vi "MKS METER - Error Handler.vi"(8 "error in (no error)":errorcluster, 10 "Channel String":string, 11 "Channel":T1(ring)) -> (0 "error out":errorcluster)   [LabVIEW 2013]
uses:
  <vilib>/Utility/error.llb/DialogType.ctl
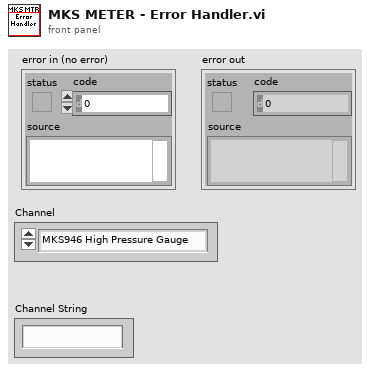
[diagram p1: front panel]
types:
  T1 = enum16{"MKS946 High Pressure Gauge", "MKS946 Separator Flow", "MKS946 Target Cavity Flow", "MKS670 Low Pressure Gauge"}
  T2 = typedef "DialogType.ctl" = u16
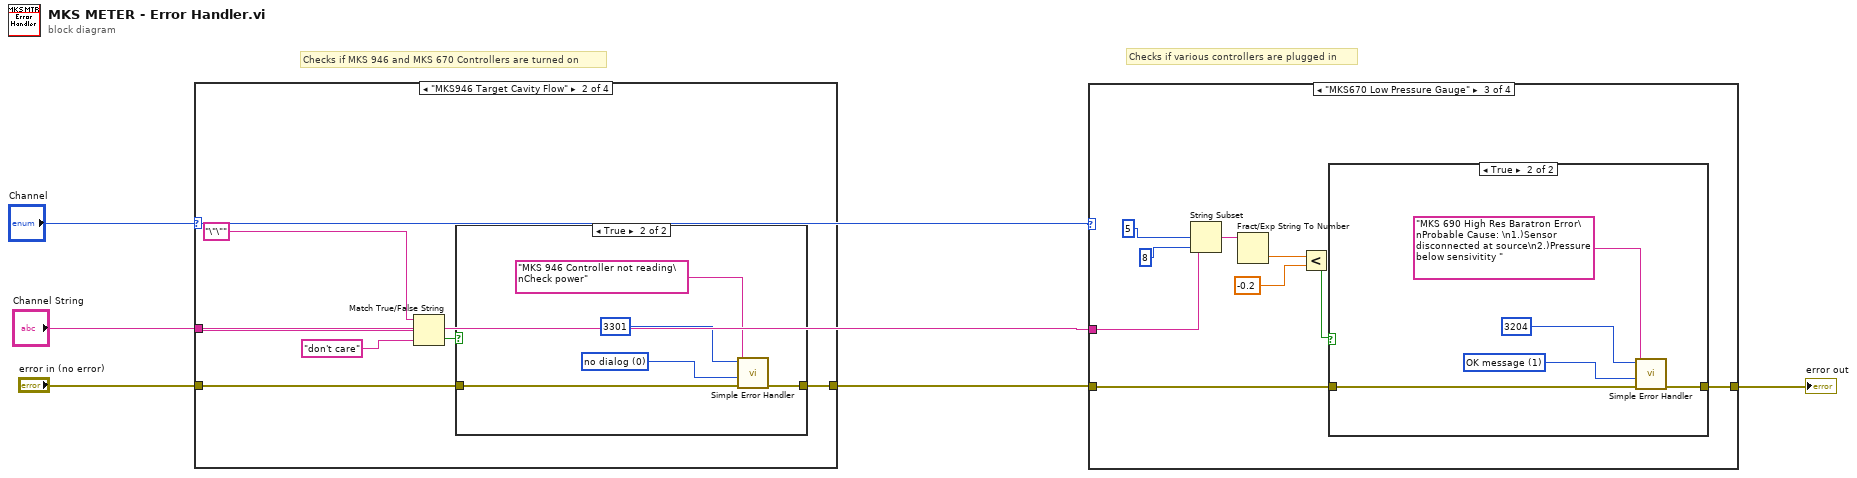
[diagram p0: block diagram]
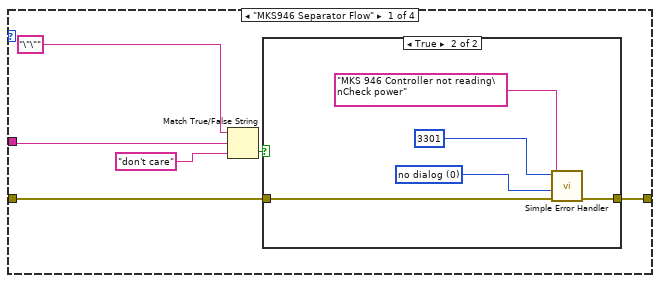
[diagram p2: hidden frame]
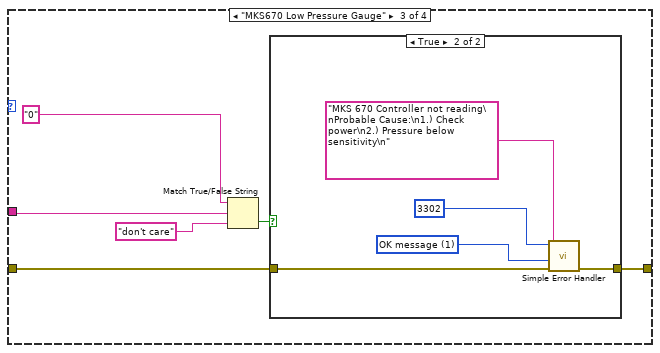
[diagram p5: hidden frame]
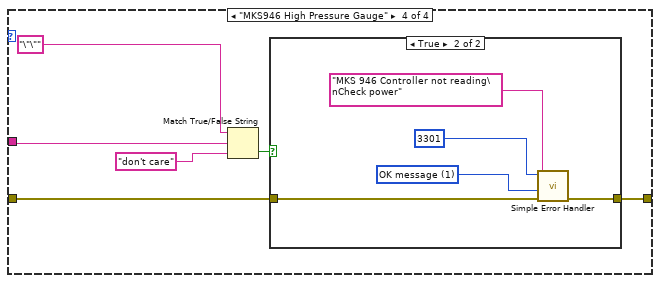
[diagram p7: hidden frame]
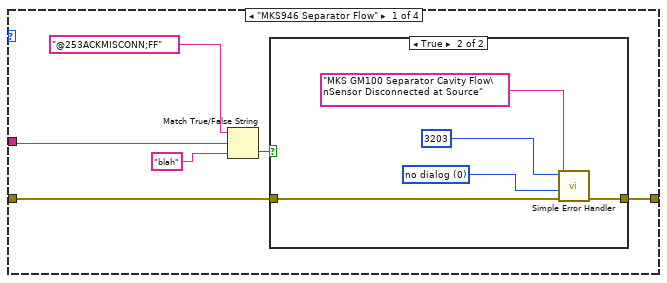
[diagram p9: hidden frame]
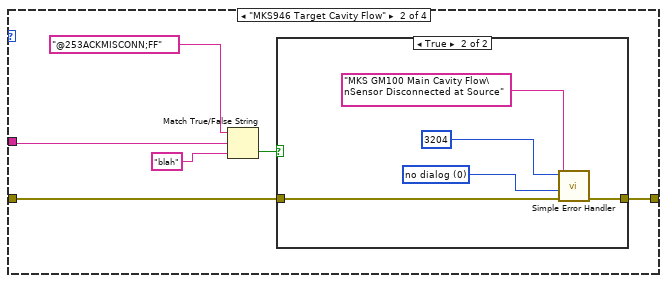
[diagram p11: hidden frame]
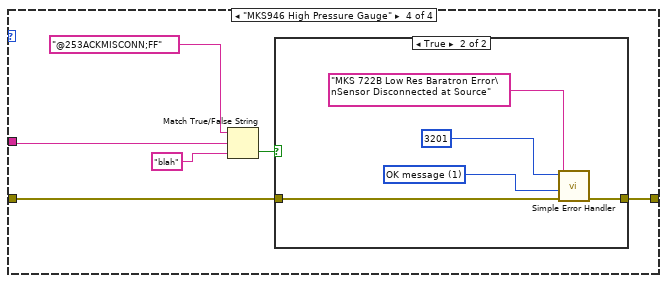
[diagram p14: hidden frame]
diagram:
  # "Checks if various controllers are plugged in"
  # "Checks if MKS 946 and MKS 670 Controllers are turned on"
  n1 = case shown="\"MKS946 Target Cavity Flow\"" "Channel" {
    tunnel: "Channel String" -> [w9 w21 w33 w45]
    tunnel: "error in (no error)" -> [w8 w20 w32 w44]
    tunnel: [w7 w19 w31 w43] -> w2
    frame "MKS946 Separator Flow" {
      n2 = Match True/False String(2:"don't care" ("output string"), 3:w9, 4:"\"\"") -> (0:w10:bool)  [unwired: 1 out]
      n3 = case shown="True" w10 {
        tunnel: w8 -> [w12 w14]
        tunnel: [w12 w13] -> w7
        frame False {
        }
        frame True {
          w17 = T2 0 items=["no dialog", "OK message", "continue or stop message", "OK message + warnings", "continue/stop + warnings"] ("type of dialog (OK msg:1)")
          n4 = call <vilib>:"Simple Error Handler.vi"("error code (no error:0)"=3301, "error source (\" \")"="MKS 946 Controller not reading\nCheck power" ("error source (\" \")"), "type of dialog (OK msg:1)"=w17, "error in (no error)"=w14) -> ("error out"=w13:errorcluster)  [unwired: 1 in, 4 out]
        }
      }
    }
    frame "MKS946 Target Cavity Flow" {
      n5 = Match True/False String(2:"don't care" ("output string"), 3:w21, 4:"\"\"") -> (0:w22:bool)  [unwired: 1 out]
      n6 = case shown="True" w22 {
        tunnel: w20 -> [w24 w26]
        tunnel: [w24 w25] -> w19
        frame False {
        }
        frame True {
          w29 = T2 0 items=["no dialog", "OK message", "continue or stop message", "OK message + warnings", "continue/stop + warnings"] ("type of dialog (OK msg:1)")
          n7 = call <vilib>:"Simple Error Handler.vi"("error code (no error:0)"=3301, "error source (\" \")"="MKS 946 Controller not reading\nCheck power" ("error source (\" \")"), "type of dialog (OK msg:1)"=w29, "error in (no error)"=w26) -> ("error out"=w25:errorcluster)  [unwired: 1 in, 4 out]
        }
      }
    }
    frame "MKS670 Low Pressure Gauge" {
      n8 = Match True/False String(2:"don't care" ("output string"), 3:w33, 4:"0") -> (0:w34:bool)  [unwired: 1 out]
      n9 = case shown="True" w34 {
        tunnel: w32 -> [w36 w38]
        tunnel: [w36 w37] -> w31
        frame False {
        }
        frame True {
          w41 = T2 1 items=["no dialog", "OK message", "continue or stop message", "OK message + warnings", "continue/stop + warnings"] ("type of dialog (OK msg:1)")
          n10 = call <vilib>:"Simple Error Handler.vi"("error code (no error:0)"=3302, "error source (\" \")"="MKS 670 Controller not reading\nProbable Cause:\n1.) Check power\n2.) Pressure below sensitivity\n" ("error source (\" \")"), "type of dialog (OK msg:1)"=w41, "error in (no error)"=w38) -> ("error out"=w37:errorcluster)  [unwired: 1 in, 4 out]
        }
      }
    }
    frame "MKS946 High Pressure Gauge" {
      n11 = Match True/False String(2:"don't care" ("output string"), 3:w45, 4:"\"\"") -> (0:w46:bool)  [unwired: 1 out]
      n12 = case shown="True" w46 {
        tunnel: w44 -> [w48 w50]
        tunnel: [w48 w49] -> w43
        frame False {
        }
        frame True {
          w53 = T2 1 items=["no dialog", "OK message", "continue or stop message", "OK message + warnings", "continue/stop + warnings"] ("type of dialog (OK msg:1)")
          n13 = call <vilib>:"Simple Error Handler.vi"("error code (no error:0)"=3301, "error source (\" \")"="MKS 946 Controller not reading\nCheck power" ("error source (\" \")"), "type of dialog (OK msg:1)"=w53, "error in (no error)"=w50) -> ("error out"=w49:errorcluster)  [unwired: 1 in, 4 out]
        }
      }
    }
  }
  n14 = case shown="\"MKS670 Low Pressure Gauge\"" "Channel" {
    tunnel: "Channel String" -> [w57 w69 w81 w96]
    tunnel: w2 -> [w56 w68 w86 w95]
    tunnel: [w55 w67 w85 w94] -> w1
    frame "MKS946 Separator Flow" {
      n15 = Match True/False String(2:"blah" ("output string"), 3:w57, 4:"@253ACKMISCONN;FF") -> (0:w58:bool)  [unwired: 1 out]
      n16 = case shown="True" w58 {
        tunnel: w56 -> [w60 w62]
        tunnel: [w60 w61] -> w55
        frame False {
        }
        frame True {
          w65 = T2 0 items=["no dialog", "OK message", "continue or stop message", "OK message + warnings", "continue/stop + warnings"] ("type of dialog (OK msg:1)")
          n17 = call <vilib>:"Simple Error Handler.vi"("error code (no error:0)"=3203, "error source (\" \")"="MKS GM100 Separator Cavity Flow\nSensor Disconnected at Source" ("error source (\" \")"), "type of dialog (OK msg:1)"=w65, "error in (no error)"=w62) -> ("error out"=w61:errorcluster)  [unwired: 1 in, 4 out]
        }
      }
    }
    frame "MKS946 Target Cavity Flow" {
      n18 = Match True/False String(2:"blah" ("output string"), 3:w69, 4:"@253ACKMISCONN;FF") -> (0:w70:bool)  [unwired: 1 out]
      n19 = case shown="True" w70 {
        tunnel: w68 -> [w72 w74]
        tunnel: [w72 w73] -> w67
        frame False {
        }
        frame True {
          w77 = T2 0 items=["no dialog", "OK message", "continue or stop message", "OK message + warnings", "continue/stop + warnings"] ("type of dialog (OK msg:1)")
          n20 = call <vilib>:"Simple Error Handler.vi"("error code (no error:0)"=3204, "error source (\" \")"="MKS GM100 Main Cavity Flow\nSensor Disconnected at Source" ("error source (\" \")"), "type of dialog (OK msg:1)"=w77, "error in (no error)"=w74) -> ("error out"=w73:errorcluster)  [unwired: 1 in, 4 out]
        }
      }
    }
    frame "MKS670 Low Pressure Gauge" {
      n21 = String Subset(string=w81, offset (0)=5 ("offset"), length (rest)=8 ("offset past number")) -> (substring=w84:string)
      n22 = Fract/Exp String To Number(string=w84) -> (number=w80:dbl)  [unwired: 3 in, 1 out]
      n23 = Less?(x=w80, y=-0.2) -> (x < y?=w78:bool)
      n24 = case shown="True" w78 {
        tunnel: w86 -> [w87 w89]
        tunnel: [w87 w88] -> w85
        frame False {
        }
        frame True {
          w92 = T2 1 items=["no dialog", "OK message", "continue or stop message", "OK message + warnings", "continue/stop + warnings"] ("type of dialog (OK msg:1)")
          n25 = call <vilib>:"Simple Error Handler.vi"("error code (no error:0)"=3204, "error source (\" \")"="MKS 690 High Res Baratron Error\nProbable Cause: \n1.)Sensor disconnected at source\n2.)Pressure below sensivitity " ("error source (\" \")"), "type of dialog (OK msg:1)"=w92, "error in (no error)"=w89) -> ("error out"=w88:errorcluster)  [unwired: 1 in, 4 out]
        }
      }
    }
    frame "MKS946 High Pressure Gauge" {
      n26 = Match True/False String(2:"blah" ("output string"), 3:w96, 4:"@253ACKMISCONN;FF") -> (0:w97:bool)  [unwired: 1 out]
      n27 = case shown="True" w97 {
        tunnel: w95 -> [w99 w101]
        tunnel: [w99 w100] -> w94
        frame False {
        }
        frame True {
          w104 = T2 1 items=["no dialog", "OK message", "continue or stop message", "OK message + warnings", "continue/stop + warnings"] ("type of dialog (OK msg:1)")
          n28 = call <vilib>:"Simple Error Handler.vi"("error code (no error:0)"=3201, "error source (\" \")"="MKS 722B Low Res Baratron Error\nSensor Disconnected at Source" ("error source (\" \")"), "type of dialog (OK msg:1)"=w104, "error in (no error)"=w101) -> ("error out"=w100:errorcluster)  [unwired: 1 in, 4 out]
        }
      }
    }
  }
  "error out" <- w1
